vi "_WaitAttach.vi"(8 "error in":errorcluster, 10 "milliseconds":i32=5000, 11 "Device In":i32) -> (0 "error out":errorcluster, 3 "Device Out":i32)   [LabVIEW 2014]
uses:
  phidget21.dll
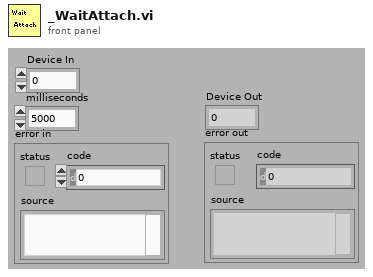
[diagram p1: front panel]
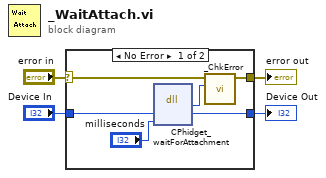
[diagram p0: block diagram]
diagram:
  n1 = case shown="No Error" "error in" {
    selector: "error in" -> [w7 w12]
    tunnel: [w5 w12] -> w3
    tunnel: [w10 w11] -> w2
    tunnel: "Device In" -> [w8 w11]
    frame No Error {
      n2 = dll-call lib="phidget21.*" fn="CPhidget_waitForAttachment"("phid"=w8, "milliseconds"="milliseconds") -> (w6:i32, "phid"=w10:i32)  [unwired: 4 in, 2 out]
      n3 = call "_ChkError.vi"("Return Code"=w6, "error in (no error)"=w7) -> ("error out"=w5:errorcluster)  [unwired: 9 in]
    }
    frame Error {
    }
  }
  "error out" <- w3
  "Device Out" <- w2
